vi "005 100 temperatures.vi"() -> ()   [LabVIEW 2019]
panel:
  out "Array":dbl[](array[numeric])
  out "Waveform Graph":cluster{i32, dbl, dbl[]}(graph)
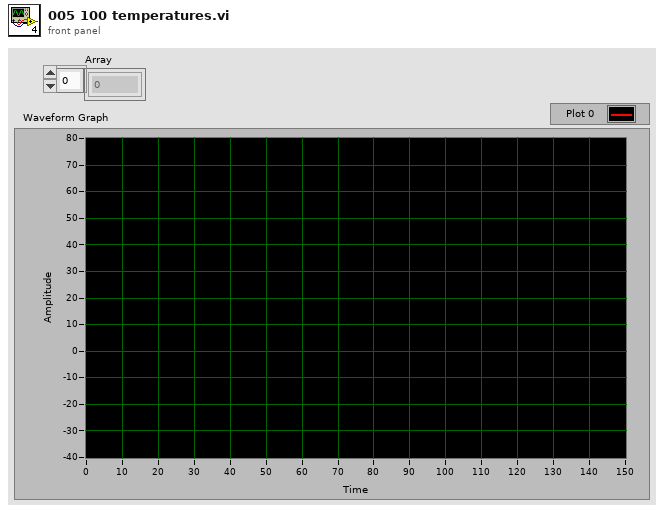
[diagram p1: front panel]
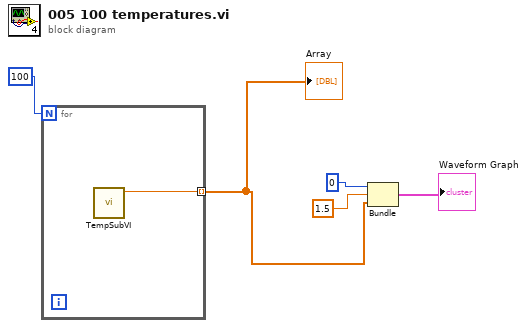
[diagram p0: block diagram]
diagram:
  n1 = for {
    N: 100 -> [_]
    tunnel: [w6] -> w1 mode=indexing
    n2 = call "TempSubVI.vi"() -> ("temp"=w6:dbl)  [unwired: 11 in]
  }
  "Array" <- w1
  n3 = Bundle(0, 1.5, w1) -> (→"Waveform Graph":cluster{i32, dbl, dbl[]})  [unwired: 1 in]
